vi "Read Mode for Deleting Stale Data.vi"(8 "error in (no error)":errorcluster, 11 "Waveforms (N Ch) in":refnum<class "Waveforms (N Ch).lvclass">) -> (0 "error out":errorcluster, 2 "delete stale samples when":T1, 3 "Waveforms (N Ch) out":refnum<class "Waveforms (N Ch).lvclass">)   [LabVIEW 2017, in "Waveforms (N Ch).lvclass"]
uses:
  <vilib>/addons/_NISVFA/_Shared subVIs/Data Objects/Waveforms (DBL)/Waveforms (N Ch).lvclass
  C:/Program Files (x86)/National Instruments/LabVIEW 2017/vi.lib/addons/_NISVFA/_Shared subVIs/Data Objects/Data/Data.lvclass
  <vilib>/addons/_NISVFA/_Shared subVIs/Controls/svc_Delete Data Options (enum).ctl
  <vilib>/addons/_NISVFA/_Shared subVIs/Data Objects/Data/Data.lvclass/Data.ctl
  <vilib>/addons/_NISVFA/_Shared subVIs/Data Objects/Data/Data.lvclass
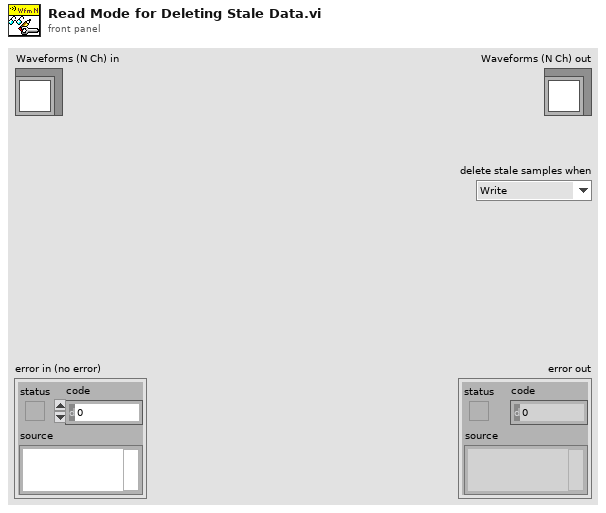
[diagram p1: front panel]
types:
  T1 = typedef "svc_Delete Data Options (enum).ctl" = enum16{"Write", "Read", "Release"}
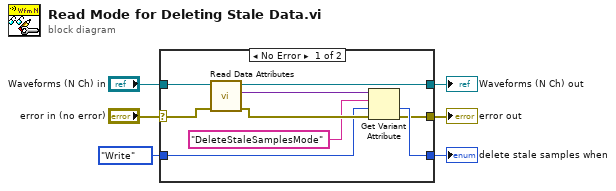
[diagram p0: block diagram]
diagram:
  n1 = case shown="No Error" "error in (no error)" {
    selector: "error in (no error)" -> [w9 w17]
    tunnel: [w8 w17] -> w5
    tunnel: [w11 w18] -> w3
    tunnel: "Waveforms (N Ch) in" -> [w12 w18]
    tunnel: [w10 w16] -> w2
    tunnel: svc_Delete_Data_Options_(enum)."Write" ("delete stale samples when") -> [w7 w16]
    frame No Error {
      n2 = call <vilib>:"Read Data Attributes.vi"("error in (no error)"=w9, "Data in"=w12) -> ("error out"=w14:errorcluster, "data attributes"=w15:variant, "Data out"=w11:refnum<class "Waveforms (N Ch).lvclass">)  [unwired: 7 in]
      n3 = Get Variant Attribute(Variant=w15, name="DeleteStaleSamplesMode", default value (empty Variant)=w7, error in=w14) -> (value=w10:T1, error out=w8:errorcluster)  [unwired: 2 out]
    }
    frame Error {
    }
  }
  "error out" <- w5
  "Waveforms (N Ch) out" <- w3
  "delete stale samples when" <- w2
